vi "OpenIVIsamplescope.vi"(2 "channel name (\"CHANNEL1\")":string="CHANNEL1", 3 "logical name (\"SampleScope\")":string="SampleScope") -> (0 "error out":errorcluster {"code" format="%.0x"}, 1 "instrument handle out":refnum<k15>)   [LabVIEW 2013]
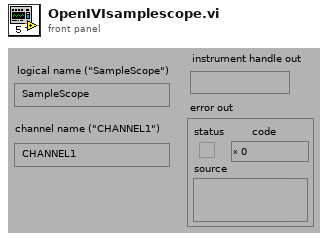
[diagram p1: front panel]
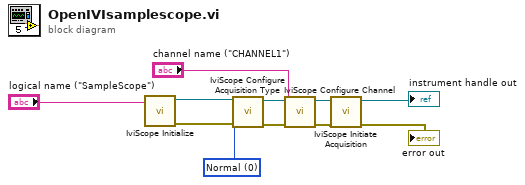
[diagram p0: block diagram]
diagram:
  w7 = 0 items=["Normal", "Peak Detect", "High Resolution", "Envelope", "Average"] ("acquisition type (Normal)")
  n1 = call <vilib>:"IviScope Initialize.vi"("logical name (\"SampleScope\")"="logical name (\"SampleScope\")") -> ("error out"=w6:errorcluster, "instrument handle out"=w5:refnum<k15>)  [unwired: 3 in, 6 out]
  n2 = call <vilib>:"IviScope Configure Acquisition Type.vi"("error in (no error)"=w6, "acquisition type (Normal)"=w7, "instrument handle"=w5) -> ("error out"=w9:errorcluster, "instrument handle out"=w11:refnum<k15>)  [unwired: 7 out]
  n3 = call <vilib>:"IviScope Configure Channel.vi"("error in (no error)"=w9, "channel name (\"CHANNEL1\")"="channel name (\"CHANNEL1\")", "instrument handle"=w11) -> ("error out"=w8:errorcluster, "instrument handle out"=w10:refnum<k15>)  [unwired: 5 in, 2 out]
  n4 = call <vilib>:"IviScope Initiate Acquisition.vi"("error in (no error)"=w8, "instrument handle"=w10) -> ("error out"=→"error out":errorcluster, "instrument handle out"=→"instrument handle out":refnum<k15>)  [unwired: 8 out]
